vi "initialise.vi"(8 "error in (no error)":errorcluster, 11 "DL090202ScanHead in":refnum<class "ScanHeadDL090202.lvclass">) -> (0 "error out":errorcluster, 3 "DL090202ScanHead out":refnum<class "ScanHeadDL090202.lvclass">)   [LabVIEW 2010, in "ScanHeadDL090202.lvclass"]
doc: "The dynamic dispatch-version of this VI initalises the plug-in object by allocating and initalising any dynamic resources need."
uses:
  ScanHeadDL090202.lvclass
  GenericScanHead/GenericScanHead/GenericScanHead.lvclass
  ScanHeadDL090202.lvclass/ScanHeadDL090202.ctl
  DigitalOut/GenericDigitalOut/GenericDigitalOut/GenericDigitalOut.lvclass
  Clock/GenericClock/GenericClock/GenericClock.lvclass
  common/classes/ErrorController/ErrorController/class_data.vi
  common/classes/ErrorController/ErrorController/ErrorController.lvclass
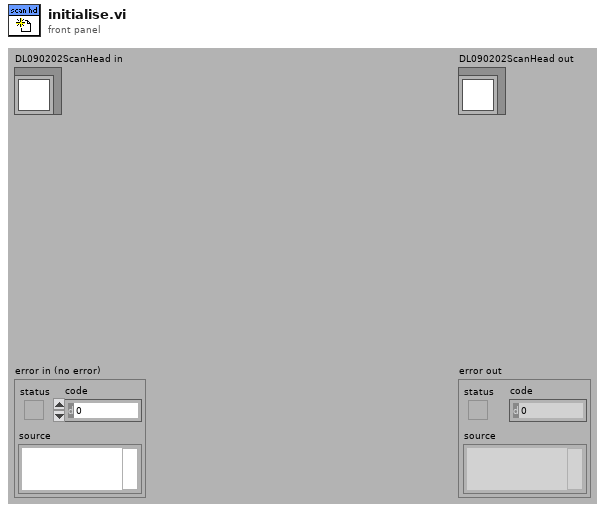
[diagram p1: front panel]
types:
  T1 = enum8{"Enabled", "Disabled", "Disabled and Grayed Out"}
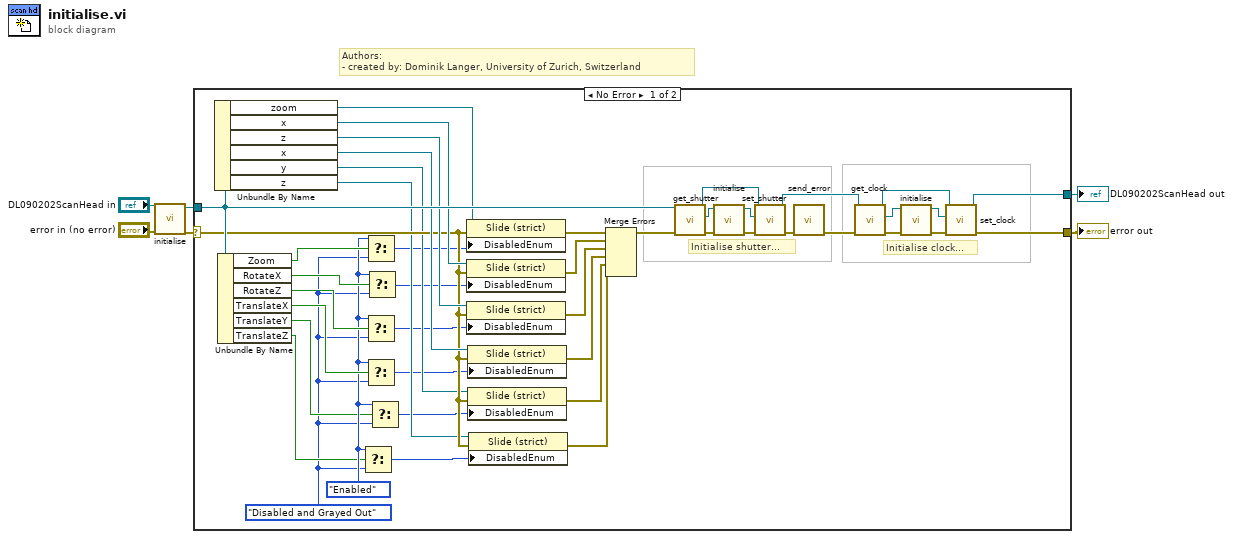
[diagram p0: block diagram]
diagram:
  # "Authors: \n- created by: Dominik Langer, University of Zurich, Switzerland"
  n1 = call-parent "initialise.vi"("error in (no error)"="error in (no error)", "GenericPlugin in"="DL090202ScanHead in") -> ("error out"=w4:errorcluster, "GenericPlugin out"=w3:refnum<class "ScanHeadDL090202.lvclass">)  [unwired: 8 out]
  n2 = case shown="No Error" w4 {
    selector: w4 -> [w40 w51]
    tunnel: w3 -> [w45 w52]
    tunnel: [w7 w51] -> w2
    tunnel: [w8 w52] -> w1
    frame No Error {
      w22 = T1."Disabled and Grayed Out" ("Disabled")
      w25 = T1."Enabled" ("Disabled")
      # "Initialise clock..."
      # "Initialise shutter..."
      n3 = Unbundle By Name(w45) -> ("zoom"=w44:refnum<vi>, "x"=w43:refnum<vi>, "z"=w42:refnum<vi>, "x"=w41:refnum<vi>, "y"=w39:refnum<vi>, "z"=w38:refnum<vi>)
      n4 = Unbundle By Name(w45) -> ("Zoom"=w35:bool, "RotateX"=w34:bool, "RotateZ"=w33:bool, "TranslateX"=w28:bool, "TranslateY"=w24:bool, "TranslateZ"=w23:bool)
      n5 = Select(t=w25, s=w23, f=w22) -> (s? t:f=w26:T1)
      n6 = Select(t=w25, s=w35, f=w22) -> (s? t:f=w32:T1)
      n7 = Select(t=w25, s=w33, f=w22) -> (s? t:f=w30:T1)
      n8 = Select(t=w25, s=w28, f=w22) -> (s? t:f=w29:T1)
      n9 = Select(t=w25, s=w34, f=w22) -> (s? t:f=w31:T1)
      n10 = Select(t=w25, s=w24, f=w22) -> (s? t:f=w27:T1)
      n11 = property class="Slide (strict)"(reference=w44, error in=w40, "DisabledEnum"=w32) -> (error out=w37:errorcluster)  [unwired: 1 out]
      n12 = property class="Slide (strict)"(reference=w43, error in=w40, "DisabledEnum"=w31) -> (error out=w21:errorcluster)  [unwired: 1 out]
      n13 = property class="Slide (strict)"(reference=w42, error in=w40, "DisabledEnum"=w30) -> (error out=w20:errorcluster)  [unwired: 1 out]
      n14 = property class="Slide (strict)"(reference=w41, error in=w40, "DisabledEnum"=w29) -> (error out=w19:errorcluster)  [unwired: 1 out]
      n15 = property class="Slide (strict)"(reference=w39, error in=w40, "DisabledEnum"=w27) -> (error out=w18:errorcluster)  [unwired: 1 out]
      n16 = property class="Slide (strict)"(reference=w38, error in=w40, "DisabledEnum"=w26) -> (error out=w17:errorcluster)  [unwired: 1 out]
      n17 = Merge Errors(w37, w21, w20, w19, w18, w17) -> (w36:errorcluster)
      n18 = call-dynamic "get_shutter.vi"("error in (no error)"=w36, "DL090202ScanHead.lvclass in"=w45) -> ("error out"=w47:errorcluster, "GenericDigitalOut.lvclass"=w46:refnum<class "GenericDigitalOut.lvclass">, "DL090202ScanHead.lvclass out"=w50:refnum<class "ScanHeadDL090202.lvclass">)  [unwired: 7 out]
      n19 = call-dynamic "initialise.vi"("error in (no error)"=w47, "GenericPlugin in"=w46) -> ("error out"=w48:errorcluster, "GenericPlugin out"=w49:refnum<class "GenericDigitalOut.lvclass">)  [unwired: 8 out]
      n20 = call-dynamic "set_shutter.vi"("error in (no error)"=w48, "GenericDigitalOut.lvclass"=w49, "DL090202ScanHead.lvclass in"=w50) -> ("error out"=w16:errorcluster, "DL090202ScanHead.lvclass out"=w9:refnum<class "ScanHeadDL090202.lvclass">)  [unwired: 7 out]
      n21 = call "send_error.vi"("error in (no error)"=w16) -> ("error out"=w11:errorcluster)  [unwired: 10 in]
      n22 = call-dynamic "get_clock.vi"("error in (no error)"=w11, "DL090202ScanHead.lvclass in"=w9) -> ("error out"=w15:errorcluster, "GenericClock.lvclass"=w13:refnum<class "GenericClock.lvclass">, "DL090202ScanHead.lvclass out"=w10:refnum<class "ScanHeadDL090202.lvclass">)  [unwired: 7 out]
      n23 = call-dynamic "initialise.vi"("error in (no error)"=w15, "GenericPlugin in"=w13) -> ("error out"=w14:errorcluster, "GenericPlugin out"=w12:refnum<class "GenericClock.lvclass">)  [unwired: 8 out]
      n24 = call-dynamic "set_clock.vi"("error in (no error)"=w14, "GenericClock.lvclass"=w12, "DL090202ScanHead.lvclass in"=w10) -> ("error out"=w7:errorcluster, "DL090202ScanHead.lvclass out"=w8:refnum<class "ScanHeadDL090202.lvclass">)  [unwired: 7 out]
    }
    frame Error {
    }
  }
  "error out" <- w2
  "DL090202ScanHead out" <- w1
